vi "Close_BK9201.vi"(2 "error in (no error)":errorcluster, 3 "Instrument In":refnum<visa-resource-name>) -> (0 "error out":errorcluster)   [LabVIEW 2023]
uses:
  <instrlib>/BK Precision 9200 Series/BK Precision 9200 Series.lvlib
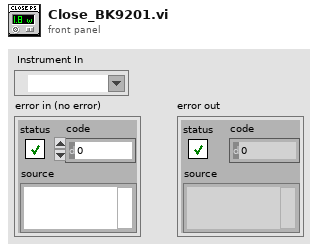
[diagram p1: front panel]
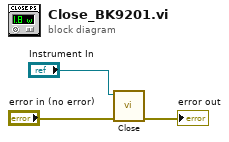
[diagram p0: block diagram]
diagram:
  n1 = call <instrlib>:"Close.vi"("error in (no error)"="error in (no error)", "VISA resource name"="Instrument In") -> ("error out"=→"error out":errorcluster)  [unwired: 9 in]
